vi "SECoP-filterStoredCommand.vi"(8 "error in (no error)":errorcluster, 9 "filter action":T1, 10 "filter accessibles":string[](array[string]), 11 "DLL path (in)":T3) -> (0 "error out":errorcluster, 1 "SECoP_data":T2 {"ptr64" format="%.0x"; "ptr32" format="%.0x"}, 2 "command/parameter path":string, 3 "DLL path (out)":T3, 4 "action":T1, 5 "command id":u64)   [LabVIEW 2023, in "SECoP.lvlib"]
doc: "Call <b>\"SECoP-filterStoredCommand.vi\"</b> regulary to check, if there is something to do for selected accessibles only. If yes, it will return successfully with an id, what to do, a parameter/command name and new set value or argument.\n\n<b>Note</b>: Keep in mind, that this will filter out only selected accessibles. If there are others, they have to handled with their own filter or use \"SECoP-getStoredCommand.vi\".\n\n<b>DLL path</b> input and output of cluster from \"SECoP-Initialize.vi\"\n<b>filter accessibles</b> string list of selected accessibles including node id and module name (format <b>node-id:module:accessible</b>)\n<b>filter action</b> selected action type: <b>any</b> (read/change/do) or special action type\n<b>command id</b> on match: command id for \"SECoP-putCommandAnswer.vi\"\n<b>action id</b> on match: action id to handle\n<b>command/parameter path</b> on match: full name of accessible\n<b>SECoP_data</b> on match with change or do: input data from SECoP-client"
uses:
  SECoP.lvlib
  SECoP-libraries.ctl
  SECoP-action.ctl
  SECoP-data/SECoP-data.ctl
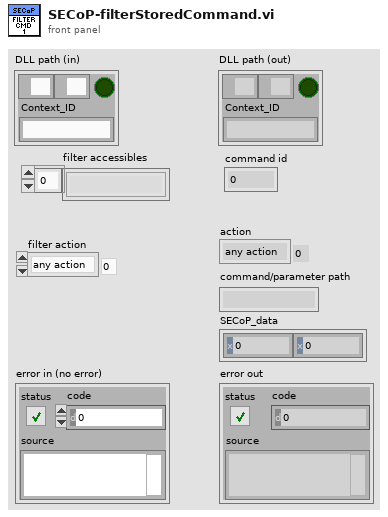
[diagram p1: front panel]
types:
  T1 = typedef "SECoP.lvlib/SECoP-action.ctl" = enum32{"any action", "read", "change", "do cmd"}
  T2 = typedef "SECoP.lvlib/SECoP-data.ctl" = cluster{"ptr32":u32, "ptr64":u64}
  T3 = typedef "SECoP.lvlib/SECoP-libraries.ctl" = cluster{"serverDLL":path, "variantDLL":path, "cleanup_mode":bool, "Context_ID":string}
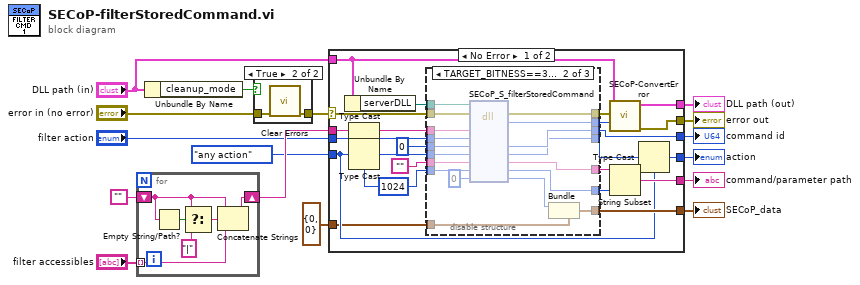
[diagram p0: block diagram]
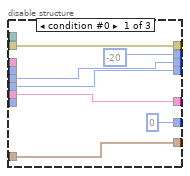
[diagram p3: hidden frame]
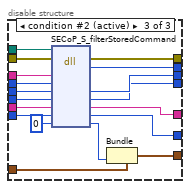
[diagram p4: hidden frame]
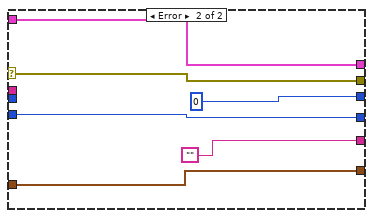
[diagram p5: hidden frame]
diagram:
  n1 = for {
    shift-right: [w17] -> w16
    shift-left: "" -> [w20]
    tunnel: "filter accessibles" -> [w18] mode=indexing
    n2 = Empty String/Path?(string/path=w20) -> (empty?=w22:bool)
    n3 = Select(t=w20, s=w22, f="|") -> (s? t:f=w21:string)
    n4 = Concatenate Strings(w20, w21, w18) -> (w17:string)
  }
  n5 = Unbundle By Name("DLL path (in)") -> ("cleanup_mode"=w11:bool)
  n6 = case shown="True" w11 {
    tunnel: "error in (no error)" -> [w23 w25]
    tunnel: [w23 w24] -> w9
    frame False {
    }
    frame True {
      n7 = call <vilib>:"Clear Errors.vi"("error in (no error)"=w25) -> ("error out"=w24:errorcluster)  [unwired: 5 in, 1 out]
    }
  }
  n8 = case shown="No Error" w9 {
    selector: w9 -> [w46 w96]
    tunnel: "DLL path (in)" -> [w31 w97]
    tunnel: [w47 w97] -> w15
    tunnel: [w48 w96] -> w14
    tunnel: [w39 i64 0 ("id")] -> w13
    tunnel: [w36 w94] -> w7
    tunnel: [w37 ""] -> w12
    tunnel: SECoP-action."any action" ("SECoP_action") -> [w34 w94]
    tunnel: [w35 w92] -> w5
    tunnel: T2 {"ptr32"=0, "ptr64"=0} ("SECoP_data") -> [w32 w92]
    tunnel: w16 -> [w29 _]
    tunnel: "filter action" -> [w26 _]
    frame No Error {
      w27 = 1024
      n9 = Unbundle By Name(w31) -> ("serverDLL"=w30:path)
      n10 = Type Cast(type=w27, x=w26) -> (*(type *) &x=w28:i32)
      n11 = Type Cast(type=w27, x=w34) -> (*(type *) &x=w33:i32)
      n12 = disable-structure shown="TARGET_BITNESS==32" {
        disable-tunnel: w46 -> [w55 w73 w86]
        disable-tunnel: w30 -> [_ w72 w91]
        disable-tunnel: [w55 w71 w85] -> w45
        disable-tunnel: [-20 ("return type") w70 w84] -> w44
        disable-tunnel: u64 0 ("id") -> [w52 w69 w87]
        disable-tunnel: "" -> [w50 w68 w89]
        disable-tunnel: w27 -> [_ w67 w90]
        disable-tunnel: [0 ("parameter size") w66 w80] -> w41
        disable-tunnel: [w50 w65 w81] -> w40
        disable-tunnel: [w52 w64 w83] -> w39
        disable-tunnel: [w51 w63 w82] -> w38
        disable-tunnel: w33 -> [w51 w62 w88]
        disable-tunnel: [w53 w61 w77] -> w35
        disable-tunnel: w32 -> [w53 w60 w79]
        disable-tunnel: w29 -> [_ w57 w74]
        disable-tunnel: w28 -> [_ w56 w75]
        frame condition #0 {
        }
        frame condition #1 {
          n13 = dll-call lib="Z:/Praktische Aufgaben/SECoP-LabVIEW2015/32bit/SECoP32.dll" fn="SECoP_S_filterStoredCommand"(path in=w72, error in=w73, "szFilterAccessibles"=w57, "iFilterAction"=w56, "pllId"=w69, "piAction"=w62, "szAccessible"=w68, "piAccessibleSize"=w67, "pValue"=u32 0 ("value")) -> (error out=w71:errorcluster, "return type"=w70:i32, "pllId"=w64:u64, "piAction"=w63:i32, "szAccessible"=w65:string, "piAccessibleSize"=w66:i32, "pValue"=w59:u32)  [unwired: 3 in, 1 out]
          n14 = Bundle(cluster=w60, "ptr32"=w59) -> (w61:T2)  [unwired: 1 in]
        }
        frame condition #2 (active) {
          n15 = dll-call lib="Z:/Praktische Aufgaben/SECoP-LabVIEW2015/32bit/SECoP32.dll" fn="SECoP_S_filterStoredCommand"(path in=w91, error in=w86, "szFilterAccessibles"=w74, "iFilterAction"=w75, "pllId"=w87, "piAction"=w88, "szAccessible"=w89, "piAccessibleSize"=w90, "pValue"=u64 0 ("value")) -> (error out=w85:errorcluster, "return type"=w84:i32, "pllId"=w83:u64, "piAction"=w82:i32, "szAccessible"=w81:string, "piAccessibleSize"=w80:i32, "pValue"=w78:u64)  [unwired: 3 in, 1 out]
          n16 = Bundle(cluster=w79, "ptr64"=w78) -> (w77:T2)  [unwired: 1 in]
        }
      }
      n17 = call "SECoP-ConvertError.vi"("return code"=w44, "error in (no error)"=w45, "DLL path (in)"=w31) -> ("error out"=w48:errorcluster, "DLL path (out)"=w47:T3)  [unwired: 7 in]
      n18 = String Subset(string=w40, length (rest)=w41) -> (substring=w37:string)  [unwired: 1 in]
      n19 = Type Cast(type=w34, x=w38) -> (*(type *) &x=w36:T1)
    }
    frame Error {
    }
  }
  "DLL path (out)" <- w15
  "error out" <- w14
  "command/parameter path" <- w12
  "command id" <- w13
  "action" <- w7
  "SECoP_data" <- w5
